vi "Plugin.Rx.vi"(8 "error in (no error)":errorcluster, 10 "Transfer Group in":refnum<class "DSF.Engine.Transfer Group.lvclass">, 11 "UDP Plugin in":refnum<class "UDP Plugin.lvclass">) -> (0 "error out":errorcluster, 2 "Transfer Group out":refnum<class "DSF.Engine.Transfer Group.lvclass">, 3 "UDP Plugin out":refnum<class "UDP Plugin.lvclass">)   [LabVIEW 2017, in "UDP Plugin.lvclass"]
uses:
  UDP Plugin.lvclass
  Source/Engine/Classes/Transfer/DSF.Engine.Transfer Group.lvclass
  Source/Engine/Classes/Transfer/DSF.Engine.Transfer Group.lvclass/DSF.Engine.Transfer Group.ctl
  Source/Engine/Classes/Transfer/DSF.Engine.Transfer.lvclass/DSF.Engine.Transfer.ctl
  UDP Plugin.lvclass/UDP Plugin.ctl
  Source/Engine/Classes/Transfer/DSF.Engine.Transfer.lvclass
  Source/Engine/Classes/Buffer/DSF.Engine.Memory.Buffer.lvclass
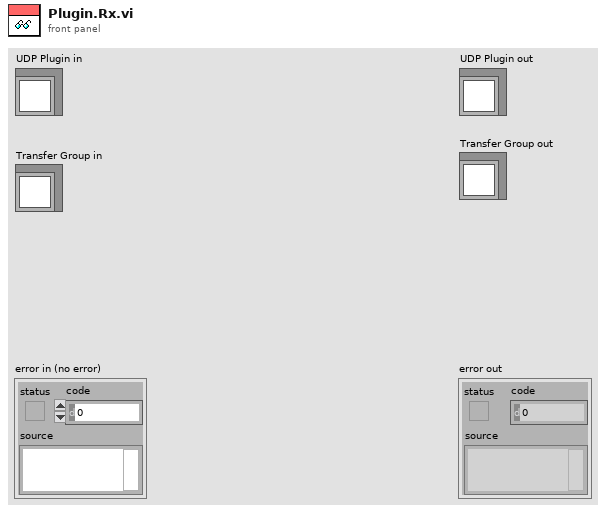
[diagram p1: front panel]
types:
  T1 = typedef "DSF.Engine.lvlib/DSF.Engine.Typedefs.ID.ctl" = i32
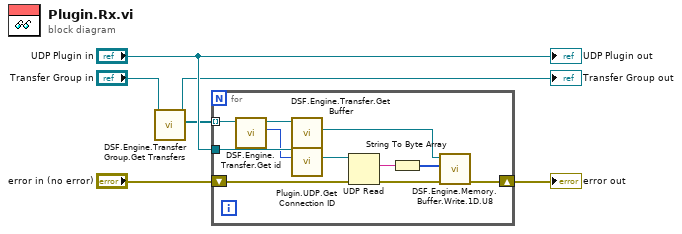
[diagram p0: block diagram]
diagram:
  n1 = call "DSF.Engine.Transfer Group.Get Transfers.vi"("Transfer Group in"="Transfer Group in") -> ("Transfers"=w2:refnum<class "DSF.Engine.Transfer.lvclass">[], "Transfer Group out"=→"Transfer Group out":refnum<class "DSF.Engine.Transfer Group.lvclass">)  [unwired: 9 in]
  n2 = for {
    tunnel: w2 -> [w17] mode=indexing
    shift-right: [w9] -> w3
    shift-left: "error in (no error)" -> [w12]
    tunnel: "UDP Plugin in" -> [w15]
    n3 = call "DSF.Engine.Transfer.Get id.vi"("Transfer in"=w17) -> ("id"=w14:T1, "Transfer out"=w16:refnum<class "DSF.Engine.Transfer.lvclass">)  [unwired: 9 in]
    n4 = call "DSF.Engine.Transfer.Get Buffer.vi"("Transfer in"=w16) -> ("Buffer"=w11:refnum<class "DSF.Engine.Memory.Buffer.lvclass">)  [unwired: 9 in, 1 out]
    n5 = call "Plugin.UDP.Get Connection ID.vi"("id"=w14, "UDP Plugin in"=w15) -> ("connection ID"=w13:refnum<k16>)  [unwired: 8 in, 1 out]
    n6 = UDP Read(connection ID=w13, 8:w12) -> (data out=w8:string, error out=w10:errorcluster)  [unwired: 2 in, 3 out]
    n7 = String To Byte Array(string=w8) -> (unsigned byte array=w7:u8[])
    n8 = call "DSF.Engine.Memory.Buffer.Write.1D.U8.vi"("error in (no error)"=w10, "buffer in"=w7, "Buffer in"=w11) -> ("error out"=w9:errorcluster)  [unwired: 5 in, 3 out]
  }
  "error out" <- w3
  "UDP Plugin out" <- "UDP Plugin in"
